vi "Main.vi"() -> ()   [LabVIEW 2017]
uses:
  <vilib>/Utility/file.llb/Read Delimited Spreadsheet (DBL).vi
  <vilib>/gmath/NI_Gmath.lvlib
  <vilib>/Analysis/NI_AALPro.lvlib
panel:
  out "Line of Fit":cluster{"Output Array":dbl[], "first row":dbl[]}(graph)
  out "Data Plot":cluster{"Output Array":dbl[], "first row":dbl[]}(graph)
  out "spread value":dbl
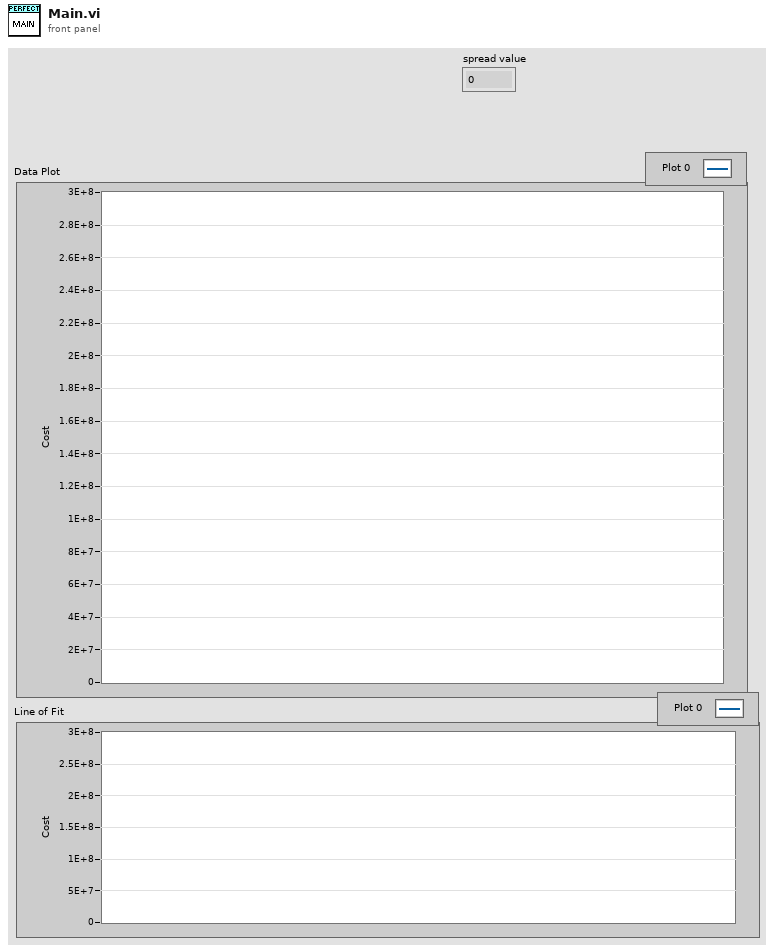
[diagram p1: front panel]
types:
  T1 = cluster{"Output Array":dbl[], "Output Array":dbl[]}
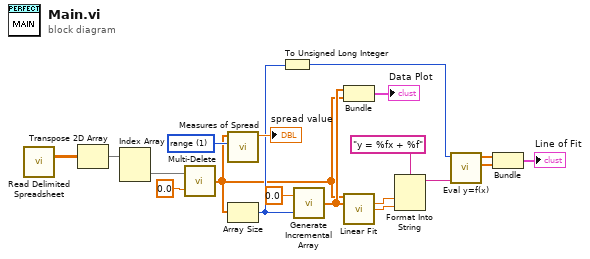
[diagram p0: block diagram]
diagram:
  w19 = 1 items=["standard deviation", "range", "mean absolute deviation", "interquartile range"] ("type")
  n1 = call-poly <vilib>:"Read Delimited Spreadsheet.vi"() -> ("all rows"=w15:dbl[][])  [unwired: 10 in, 5 out]
  n2 = Transpose 2D Array(2D array=w15) -> (transposed array=w14:dbl[][])
  n3 = Index Array(array=w14) -> (element=w4:dbl[])  [unwired: 2 in]
  n4 = call "Multi-Delete.vi"("Element to Delete"=0.0, "Input Array"=w4) -> ("Output Array"=w2:dbl[])
  n5 = call <vilib>:"Measures of Spread.vi"("type"=w19, "x array"=w2) -> ("spread value"=→"spread value":dbl)  [unwired: 8 in, 1 out]
  n6 = Array Size(array=w2) -> (size(s)=w8:i32)
  n7 = To Unsigned Long Integer(number=w8) -> (unsigned 32bit integer=w9:u32)
  n8 = call "Generate Incremental Array.vi"("Array Size"=w8, "Starting Element"=0.0) -> ("Output Array"=w16:dbl[])
  n9 = Bundle("Output Array"=w16, "Output Array"=w2) -> (→"Data Plot":T1)  [unwired: 1 in]
  n10 = call <vilib>:"Linear Fit.vi"("Y"=w2, "X"=w16) -> ("slope"=w12:dbl, "intercept"=w11:dbl)  [unwired: 9 in, 3 out]
  n11 = Format Into String(format string="y = %fx + %f", w12, w11) -> (resulting string=w10:string)  [unwired: 2 in, 1 out]
  n12 = call <vilib>:"Eval y=f(x).vi"("formula"=w10, "number of points"=w9) -> ("Y Values"=w5:dbl[], "X Values"=w6:dbl[])  [unwired: 2 in, 2 out]
  n13 = Bundle("X Values"=w6, "Y Values"=w5) -> (→"Line of Fit":cluster{"X Values":dbl[], "Y Values":dbl[]})  [unwired: 1 in]
